vi "Pre Launch Init.vi"(11 "Root Actor in":refnum<class "Root Actor.lvclass">) -> (0 "error out":errorcluster, 3 "Root Actor out":refnum<class "Root Actor.lvclass">)   [LabVIEW 2020, in "Nested Actor.lvlib" / "Root Actor.lvclass"]
doc: "(<B>Filename</B>: Actor Framework.lvlib:Actor.lvclass:Pre Launch Init.vi)\n\nDefines behavior that occurs after the Launch Nested Actor method is invoked but before the actor's Actor Core method begins running.\n\nBy default, this method does nothing. A descendant class may override it to define behavior."
uses:
  Root Actor.lvclass
  Root Actor.lvclass/Root Actor.ctl
  <vilib>/ActorFramework/Actor/Actor.lvclass
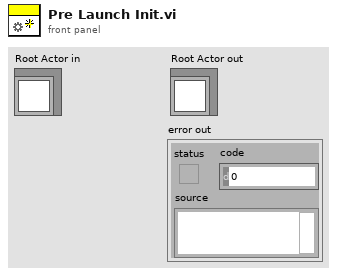
[diagram p1: front panel]
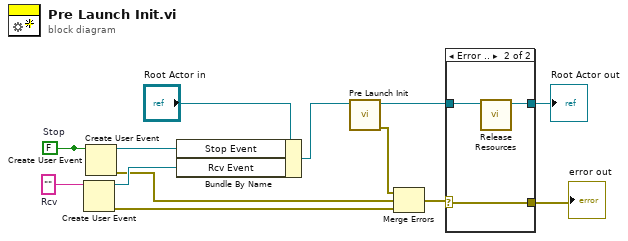
[diagram p0: block diagram]
diagram:
  w13 = ""  # Rcv
  w8 = FALSE  # Stop
  n1 = Create User Event(user event datatype=w13) -> (user event=w11:refnum<user-event>, error out=w9:errorcluster)  [unwired: 1 in]
  n2 = Create User Event(user event datatype=w8) -> (user event=w12:refnum<user-event>, error out=w10:errorcluster)  [unwired: 1 in]
  n3 = Create User Event(user event datatype=w8) -> ()  [unwired: 1 in, 2 out]
  n4 = Bundle By Name(cluster="Root Actor in", "Stop Event"=w12, "Rcv Event"=w11) -> (w6:refnum<class "Root Actor.lvclass">)
  n5 = call-parent "Pre Launch Init.vi"("Actor in"=w6) -> ("error out"=w5:errorcluster, "Actor out"=w1:refnum<class "Root Actor.lvclass">)  [unwired: 9 in]
  n6 = Merge Errors(w5, w10, w9) -> (w4:errorcluster)
  n7 = case shown="Error .." w4 {
    selector: w4 -> [w15 w16]
    tunnel: [w15 w16] -> w3
    tunnel: [w14 w17] -> w2
    tunnel: w1 -> [w14 w18]
    frame No Error {
    }
    frame Error {
      n8 = call "Release Resources.vi"("Root Actor in"=w18) -> ("Root Actor out"=w17:refnum<class "Root Actor.lvclass">)  [unwired: 10 in]
    }
  }
  "error out" <- w3
  "Root Actor out" <- w2
